vi "Ex3 RGB Image.vi"() -> ()   [LabVIEW 2020]
panel:
  in  "Color Channel":string(combo)
  out "error out":errorcluster
  out "Color Channel":T1(plugin-control)
  out "Image":T1(plugin-control)
  in  "File Path":path
  # "EX.3 RGB Image"
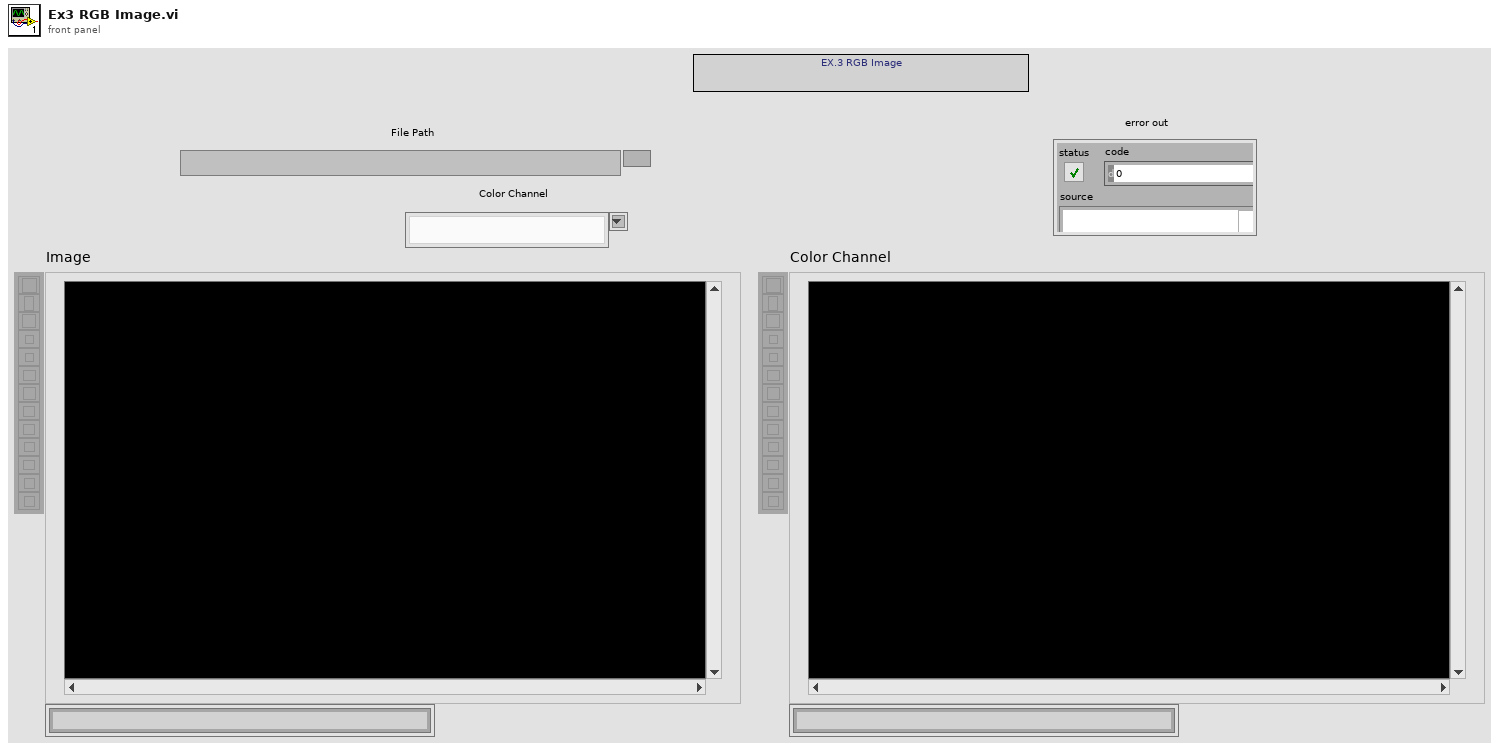
[diagram p1: front panel]
types:
  T1 = typedef "IMAQ Image.ctl" = refnum<image>
  T2 = typedef "Image Type" = u32
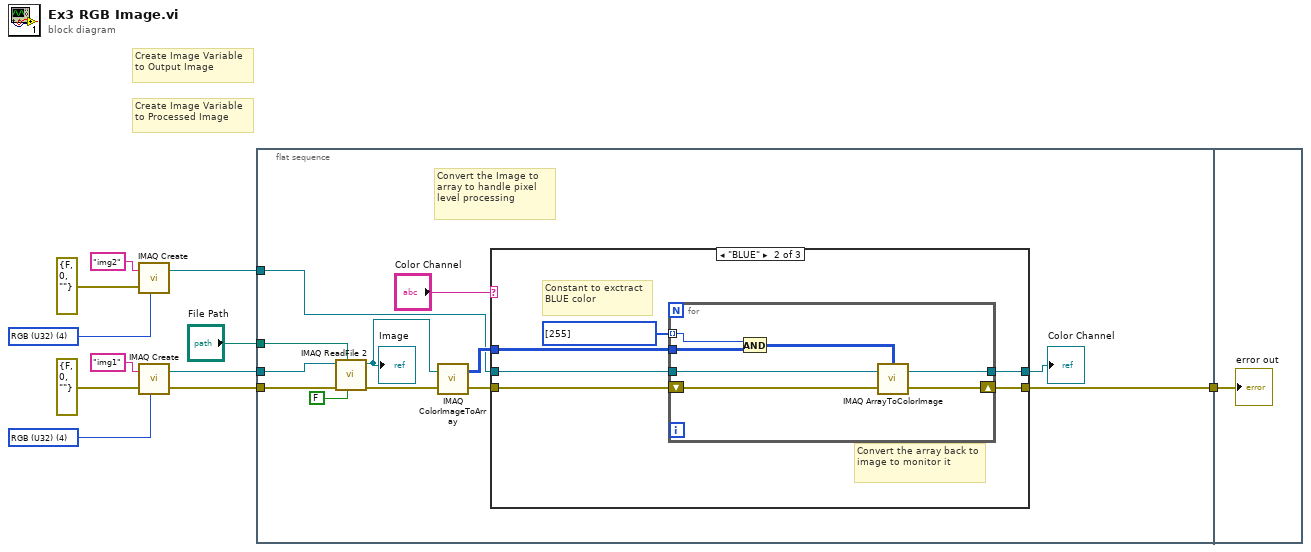
[diagram p0: block diagram]
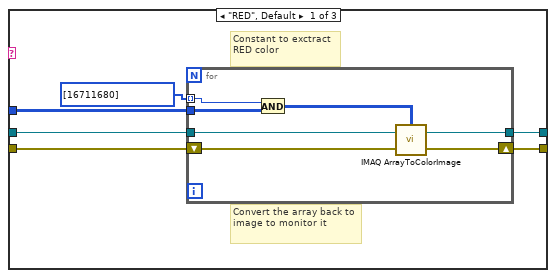
[diagram p2: hidden frame]
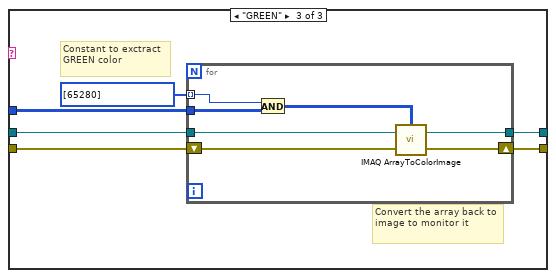
[diagram p3: hidden frame]
diagram:
  w1 = T2 4 items=["Grayscale (U8)", "Grayscale (I16)", "Grayscale (SGL)", "Complex (CSG)", "RGB (U32)", "HSL (U32)", "RGB (U64)", "Grayscale (U16)"] ("Image Type")
  w2 = T2 4 items=["Grayscale (U8)", "Grayscale (I16)", "Grayscale (SGL)", "Complex (CSG)", "RGB (U32)", "HSL (U32)", "RGB (U64)", "Grayscale (U16)"] ("Image Type")
  # "Create Image Variable to Processed Image"
  # "Create Image Variable to Output Image"
  n1 = call "IMAQ Create"("Image Name"="img2", "Image Type"=w2, "error in (no error)"=errorcluster {"status"=FALSE, "code"=0, "source"=""}) -> ("New Image"=w4:T1)  [unwired: 2 in, 1 out]
  n2 = call "IMAQ Create"("Image Name"="img1", "Image Type"=w1, "error in (no error)"=errorcluster {"status"=FALSE, "code"=0, "source"=""}) -> ("New Image"=w5:T1, "error out"=w6:errorcluster)  [unwired: 2 in]
  n3 = flat-sequence {
    tunnel: "File Path" -> [w16]
    tunnel: w6 -> [w15]
    tunnel: w5 -> [w14]
    tunnel: w4 -> [w13]
    tunnel: [w12] -> w3
    tunnel: w3 -> [w63]
    frame #0 {
      # "Convert the Image to array to handle pixel level processing"
      n4 = call "IMAQ ReadFile 2"("Use File Path Image Type"=FALSE, "File Path"=w16, "error in (no error)"=w15, "Image"=w14) -> ("error out"=w21:errorcluster, "Image Out"=w23:T1)  [unwired: 3 in, 3 out]
      "Image" <- w23
      n5 = call "IMAQ ColorImageToArray"("Image"=w23, "error in (no error)"=w21) -> ("Image Pixels (U32)"=w18:u32[][], "error out"=w19:errorcluster)  [unwired: 2 in, 1 out]
      n6 = case shown="\"BLUE\"" "Color Channel" {
        tunnel: w18 -> [w28 w39 w55]
        tunnel: w19 -> [w26 w41 w54]
        tunnel: w13 -> [w27 w40 w53]
        tunnel: [w25 w38 w51] -> w22
        tunnel: [w24 w37 w50] -> w12
        frame "RED", Default {
          # "Convert the array back to image to monitor it"
          # "Constant to exctract RED color"
          n7 = for {
            tunnel: w28 -> [w36]
            shift-right: [w33] -> w24
            shift-left: w26 -> [w34]
            tunnel: [w32] -> w25
            tunnel: w27 -> [w31]
            tunnel: i32[] [16711680] -> [w30] mode=indexing
            n8 = And(x=w30, y=w36) -> (x .and. y?=w35:u32[][])
            n9 = call "IMAQ ArrayToColorImage"("Image Pixels (U32)"=w35, "Image"=w31, "error in (no error)"=w34) -> ("Image Out"=w32:T1, "error out"=w33:errorcluster)  [unwired: 2 in]
          }
        }
        frame "BLUE" {
          # "Convert the array back to image to monitor it"
          # "Constant to exctract BLUE color"
          n10 = for {
            tunnel: w39 -> [w49]
            shift-right: [w46] -> w37
            shift-left: w41 -> [w47]
            tunnel: [w45] -> w38
            tunnel: w40 -> [w44]
            tunnel: i32[] [255] -> [w43] mode=indexing
            n11 = And(x=w43, y=w49) -> (x .and. y?=w48:u32[][])
            n12 = call "IMAQ ArrayToColorImage"("Image Pixels (U32)"=w48, "Image"=w44, "error in (no error)"=w47) -> ("Image Out"=w45:T1, "error out"=w46:errorcluster)  [unwired: 2 in]
          }
        }
        frame "GREEN" {
          # "Convert the array back to image to monitor it"
          # "Constant to exctract GREEN color"
          n13 = for {
            tunnel: w55 -> [w62]
            shift-right: [w59] -> w50
            shift-left: w54 -> [w60]
            tunnel: [w58] -> w51
            tunnel: w53 -> [w57]
            tunnel: i32[] [65280] -> [w56] mode=indexing
            n14 = And(x=w56, y=w62) -> (x .and. y?=w61:u32[][])
            n15 = call "IMAQ ArrayToColorImage"("Image Pixels (U32)"=w61, "Image"=w57, "error in (no error)"=w60) -> ("Image Out"=w58:T1, "error out"=w59:errorcluster)  [unwired: 2 in]
          }
        }
      }
      "Color Channel" <- w22
    }
    frame #1 {
      "error out" <- w63
    }
  }
